vi "waitNotifierWithTime.vi"(5 "min wait in ms (500)":u32=500, 7 "timeout in s (10)":i32=10, 8 "error in (no error)":errorcluster, 10 "Ignore case (F)":bool, 11 "Notifier in":refnum<notifier>) -> (0 "error out":errorcluster, 2 "notification":string, 3 "notifier out":refnum<notifier>)   [LabVIEW 2023]
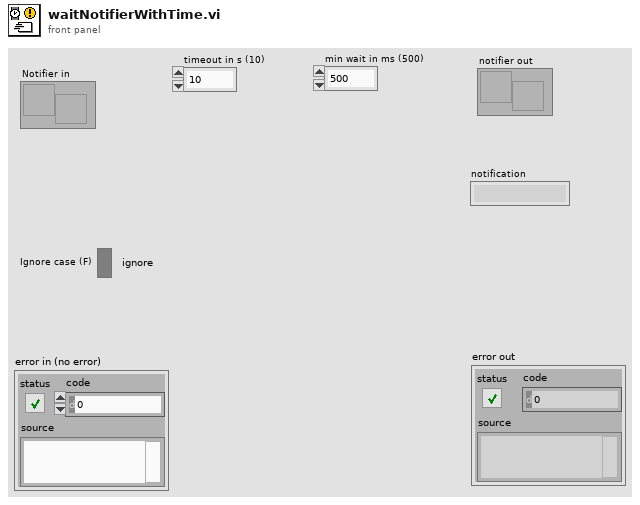
[diagram p1: front panel]
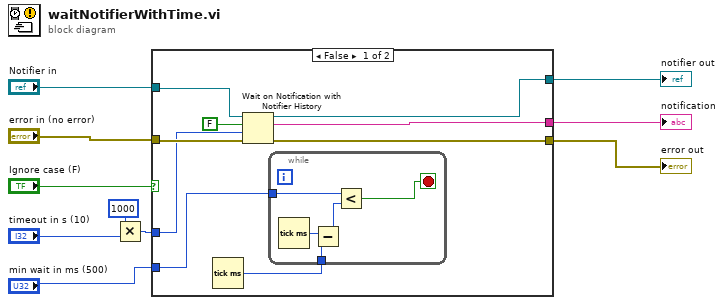
[diagram p0: block diagram]
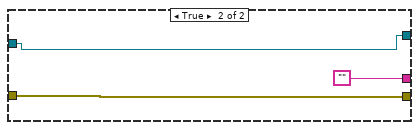
[diagram p2: hidden frame]
diagram:
  n1 = Multiply(x=1000 ("y"), y="timeout in s (10)") -> (x*y=w7:i32)
  n2 = case shown="False" "Ignore case (F)" {
    tunnel: "error in (no error)" -> [w19 w27]
    tunnel: [w18 w27] -> w9
    tunnel: "Notifier in" -> [w16 w25]
    tunnel: w7 -> [w14 _]
    tunnel: "min wait in ms (500)" -> [w13 _]
    tunnel: [w12 ""] -> w4
    tunnel: [w11 w25] -> w1
    frame False {
      n3 = Tick Count (ms)() -> (millisecond timer value=w15:u32)
      n4 = Wait on Notification with Notifier History(0:w16, 1:FALSE ("ignore previous (F)"), 2:w14, 3:w19) -> (8:w11:refnum<notifier>, 9:w12:string, 11:w18:errorcluster)  [unwired: 1 out]
      n5 = while {
        tunnel: w15 -> [w24]
        tunnel: w13 -> [w22]
        stop <- w20 stop-if-true
        n6 = Tick Count (ms)() -> (millisecond timer value=w23:u32)
        n7 = Subtract(x=w23, y=w24) -> (x-y=w21:u32)
        n8 = Less?(x=w22, y=w21) -> (x < y?=w20:bool)
      }
    }
    frame True {
    }
  }
  "error out" <- w9
  "notification" <- w4
  "notifier out" <- w1
